vi "Load Obj File.vi"() -> ()   [LabVIEW 2020, in "examples.lvlib"]
doc: "Demonstrate Loading a .Obj file with a texture."
uses:
  examples.lvlib
  ar/Create Mesh form Verticies.vi
  ar/Apply Material Information.vi
  <vilib>/Serenial/G Augmented-Reality Toolkit/g_ar_toolkit.common/Break on NILRT-ARM32.vi
  <vilib>/Utility/error.llb/Error Cluster From Error Code.vi
  <vilib>/string/Create NI GUID.vi
  <vilib>/picture/3D Picture Control/Geometries/Create Mesh.vi
  <vilib>/picture/3D Picture Control/Object/Create Object (drawable).vi
  <vilib>/picture/3D Picture Control/Object/Set Material.vi
  <vilib>/Utility/libraryn.llb/Get File Extension.vi
  <vilib>/picture/jpeg.llb/Read JPEG File.vi
  <vilib>/picture/3D Picture Control/Helpers/Apply Texture.vi
  <vilib>/picture/3D Picture Control/Helpers/Apply Texture (no reference).vi
  <vilib>/picture/png.llb/Read PNG File.vi
  <vilib>/picture/bmp.llb/Read BMP File.vi
  <vilib>/picture/3D Picture Control/Object/Create Object (name).vi
  <vilib>/picture/3D Picture Control/Object/Add Object (no reference).vi
  <vilib>/picture/3D Picture Control/Object/Add Object (reference).vi
  ar/ar.lvlib
  <vilib>/picture/3D Picture Control/NI_3D Picture Control.lvlib
panel:
  in  "Auto Focus":bool
  in  "stop":bool
  out "3D Picture":refnum<vi>(3d-picture)
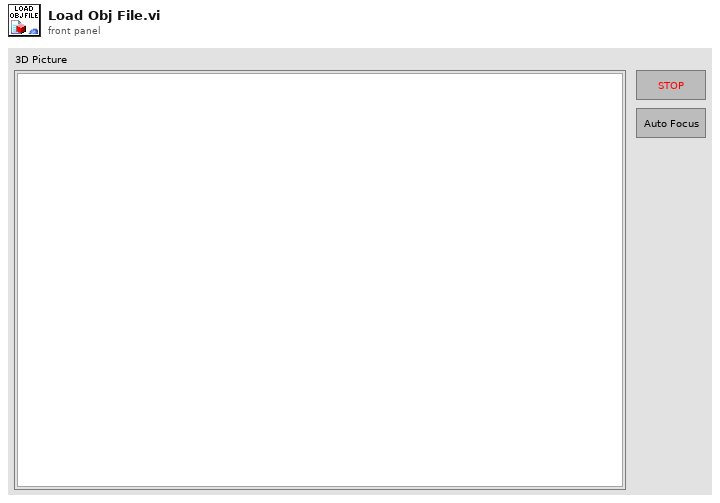
[diagram p1: front panel]
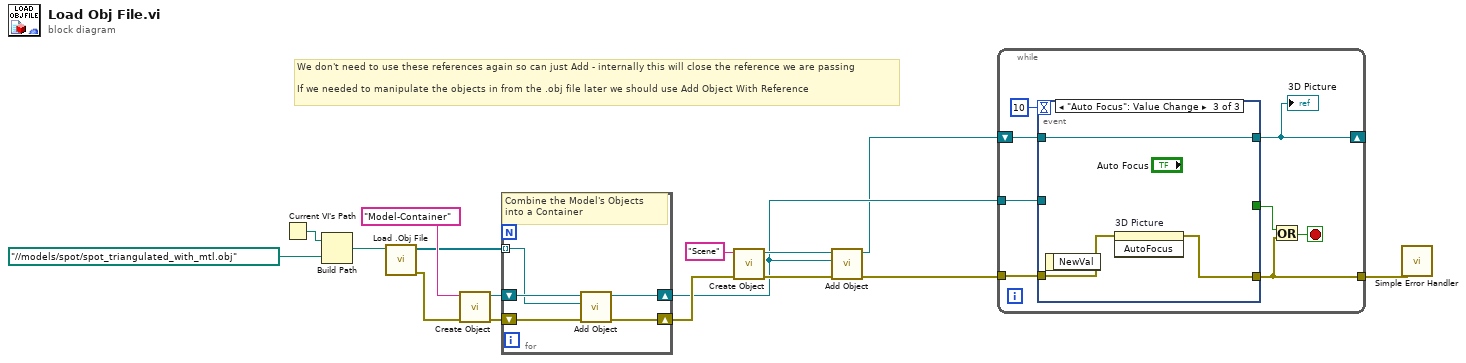
[diagram p0: block diagram]
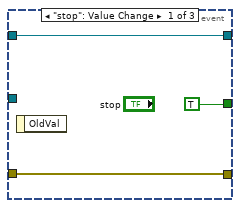
[diagram p2: hidden frame]
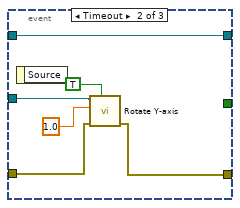
[diagram p3: hidden frame]
diagram:
  # "We don't need to use these references again so can just Add - internally this will close the reference we are passing\n\nIf we needed to manipulate the objects in from the .obj file later we should use Add Object With Reference"
  n1 = Current VI's Path() -> (path=w15:path)
  n2 = Build Path(base path=w15, name or relative path=path "../../models/spot/spot_triangulated_with_mtl.obj" ("Path")) -> (appended path=w13:path)
  n3 = call "Load .Obj File.vi"("Object Model Path"=w13) -> ("error out"=w16:errorcluster, "Objects"=w9:refnum<vi>[])  [unwired: 8 in, 1 out]
  n4 = call-poly <vilib>:"Create Object.vi"("error in (no error)"=w16, "Name"="Model-Container") -> ("error out"=w11:errorcluster, "Scene:New Object"=w10:refnum<vi>)  [unwired: 8 in]
  n5 = for {
    tunnel: w9 -> [w19] mode=indexing
    shift-right: [w18] -> w2
    shift-left: w10 -> [w20]
    shift-right: [w17] -> w6
    shift-left: w11 -> [w21]
    # "Combine the Model's Objects\ninto a Container"
    n6 = call-poly <vilib>:"Add Object.vi"("error in (no error)"=w21, "New Object In"=w19, "Scene Object In"=w20) -> ("error out"=w17:errorcluster, "Scene Object Out"=w18:refnum<vi>)  [unwired: 7 in]
  }
  n7 = call-poly <vilib>:"Create Object.vi"("error in (no error)"=w6, "Name"="Scene") -> ("error out"=w5:errorcluster, "Scene:New Object"=w7:refnum<vi>)  [unwired: 8 in]
  n8 = call-poly <vilib>:"Add Object.vi"("error in (no error)"=w5, "New Object In"=w2, "Scene Object In"=w7) -> ("error out"=w4:errorcluster, "Scene Object Out"=w1:refnum<vi>)  [unwired: 6 in, 1 out]
  n9 = while {
    tunnel: w2 -> [w29]
    tunnel: w4 -> [w27]
    tunnel: [w26] -> w3
    shift-right: [w22] -> _
    shift-left: w1 -> [w23]
    stop <- w24 stop-if-true
    n10 = event shown="[2] \"Auto Focus\": Value Change" {
      selector: _ -> [_ _ _]
      dyn-events: _ -> [_ _ _]
      timeout: 10 -> [_ _ _]
      tunnel: [TRUE _ _] -> w25
      tunnel: w29 -> [_ w38 _]
      tunnel: w27 -> [w31 w37 w40]
      tunnel: [w31 w36 w39] -> w26
      tunnel: [w30 w33 w41] -> w22
      tunnel: w23 -> [w30 w33 w41]
      event "stop": Value Change {
        n11 = event-data() -> ()  [unwired: 1 in, 1 out]
      }
      event Timeout {
        n12 = event-data() -> ()  [unwired: 1 in, 1 out]
        n13 = call <vilib>:"Rotate Y-axis.vi"("Relative?"=TRUE, "error in (no error)"=w37, "angle"=1.0, "Scene Object In"=w38) -> ("error out"=w36:errorcluster)  [unwired: 6 in, 1 out]
      }
      event "Auto Focus": Value Change {
        n14 = event-data() -> ()  [unwired: 1 in, 1 out]
        n15 = invoke on="3D Picture" class="SceneGraphDisp (strict)" method="AutoFocus"(error in=w40) -> (error out=w39:errorcluster)  [unwired: 2 in, 2 out]
      }
    }
    "3D Picture" <- w22
    n16 = Or(x=w25, y=w26) -> (x .or. y?=w24:bool)
  }
  n17 = call <vilib>:"Simple Error Handler.vi"("error in (no error)"=w3) -> ()  [unwired: 4 in, 5 out]
